vi "client.base_url.vi"(8 "error in":errorcluster, 11 "Client in":refnum<class "Client.lvclass">) -> (0 "error out":errorcluster, 2 "base url":string, 3 "Client out":refnum<class "Client.lvclass">)   [LabVIEW 2020, in "Client.lvclass"]
doc: "Returns the API address the client is connected to."
uses:
  Client.lvclass
  Client.lvclass/Client.ctl
  client.lvlib
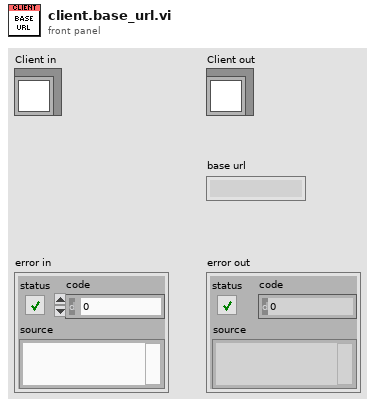
[diagram p1: front panel]
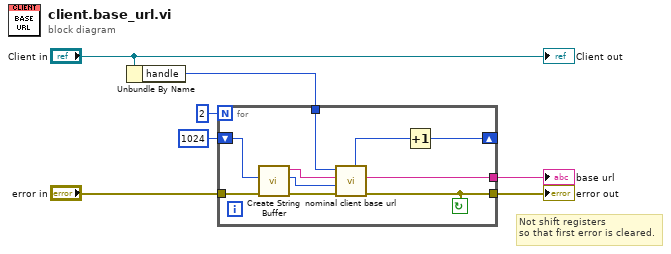
[diagram p0: block diagram]
diagram:
  # "Not shift registers\nso that first error is cleared."
  n1 = Unbundle By Name("Client in") -> ("handle"=w6:i32)
  n2 = for {
    N: 2 -> [_]
    tunnel: w6 -> [w17]
    tunnel: [w16] -> w4
    shift-right: [w8] -> _
    shift-left: 1024 ("Buffer Size (1024)") -> [w13]
    tunnel: "error in" -> [w11]
    tunnel: [w9] -> w7
    stop <- w9 continue-if-true
    n3 = call "Create String Buffer.vi"("error in"=w11, "Buffer Size (1024)"=w13) -> ("error out"=w12:errorcluster, "dub Buffer Size"=w14:i32, "String Buffer"=w15:string)  [unwired: 7 in]
    n4 = call "nominal client base url.vi"("error in (no error)"=w12, "cap"=w14, "buf"=w15, "client"=w17) -> ("error out"=w9:errorcluster, "buf out"=w16:string, "out_needed out"=w10:u32)  [unwired: 4 in, 1 out]
    n5 = Increment(x=w10) -> (x+1=w8:u32)
  }
  "error out" <- w7
  "base url" <- w4
  "Client out" <- "Client in"
